vi "Set Power Supply Output.vi"() -> ()   [LabVIEW 2020]
uses:
  lv_waveforms_toolkit.lvlib
panel:
  out "Error Out":errorcluster
  in  "stop":bool
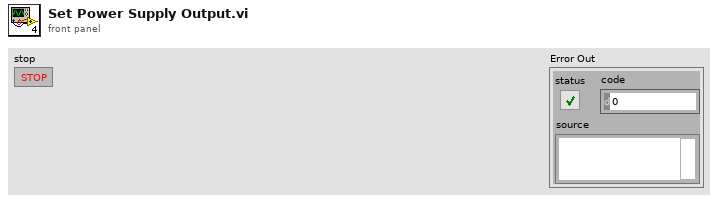
[diagram p1: front panel]
types:
  T1 = typedef "lv_waveforms_toolkit.lvlib/WFT Session.ctl" = cluster{"phdwf":i32, "Analog IO Configured":bool}
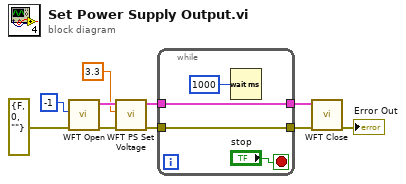
[diagram p0: block diagram]
diagram:
  n1 = call "WFT Open.vi"("Error In"=errorcluster {"status"=FALSE, "code"=0, "source"=""}, "idxDevice"=-1) -> ("Error Out"=w5:errorcluster, "WaveForms Session Out"=w6:T1)  [unwired: 7 in, 1 out]
  n2 = call "WFT PS Set Voltage.vi"("Error In"=w5, "Voltage"=3.3, "WaveForms Session In"=w6) -> ("Error Out"=w8:errorcluster, "WaveForms Session Out"=w9:T1)  [unwired: 7 in]
  n3 = while {
    tunnel: [w12] -> w10
    tunnel: w9 -> [w12]
    tunnel: w8 -> [w11]
    tunnel: [w11] -> w7
    stop <- "stop" stop-if-true
    n4 = Wait (ms)(milliseconds to wait=u32 1000) -> ()  [unwired: 1 out]
  }
  n5 = call "WFT Close.vi"("Error In"=w7, "WaveForms Session In"=w10) -> ("Error Out"=→"Error Out":errorcluster)  [unwired: 8 in, 1 out]
